vi "IP_Simulation.vi"(8 "error constant":errorcluster, 10 "Enum":T5, 11 "IP_UI":T4) -> (0 "error constant":errorcluster, 3 "Out":T4)   [LabVIEW 2021]
uses:
  Controls/IP_Cellular Tech Type def.ctl
  Controls/IP_Network_Type def.ctl
  Controls/IP_Type-Tydedef.ctl
  APIs/Controls/Base_Station_Emulator.ctl
  Controls/Enum-TypeDef.ctl
panel:
  in  "Base Station":T6
  # "Type"
  # "Network"
  # "Tech"
  # "Client Address"
  # "Throughput (Mbps)"
  # "Duration"
  # "Actions"
  # "IP-SIMULATION"
  # "ASDFADFAF"
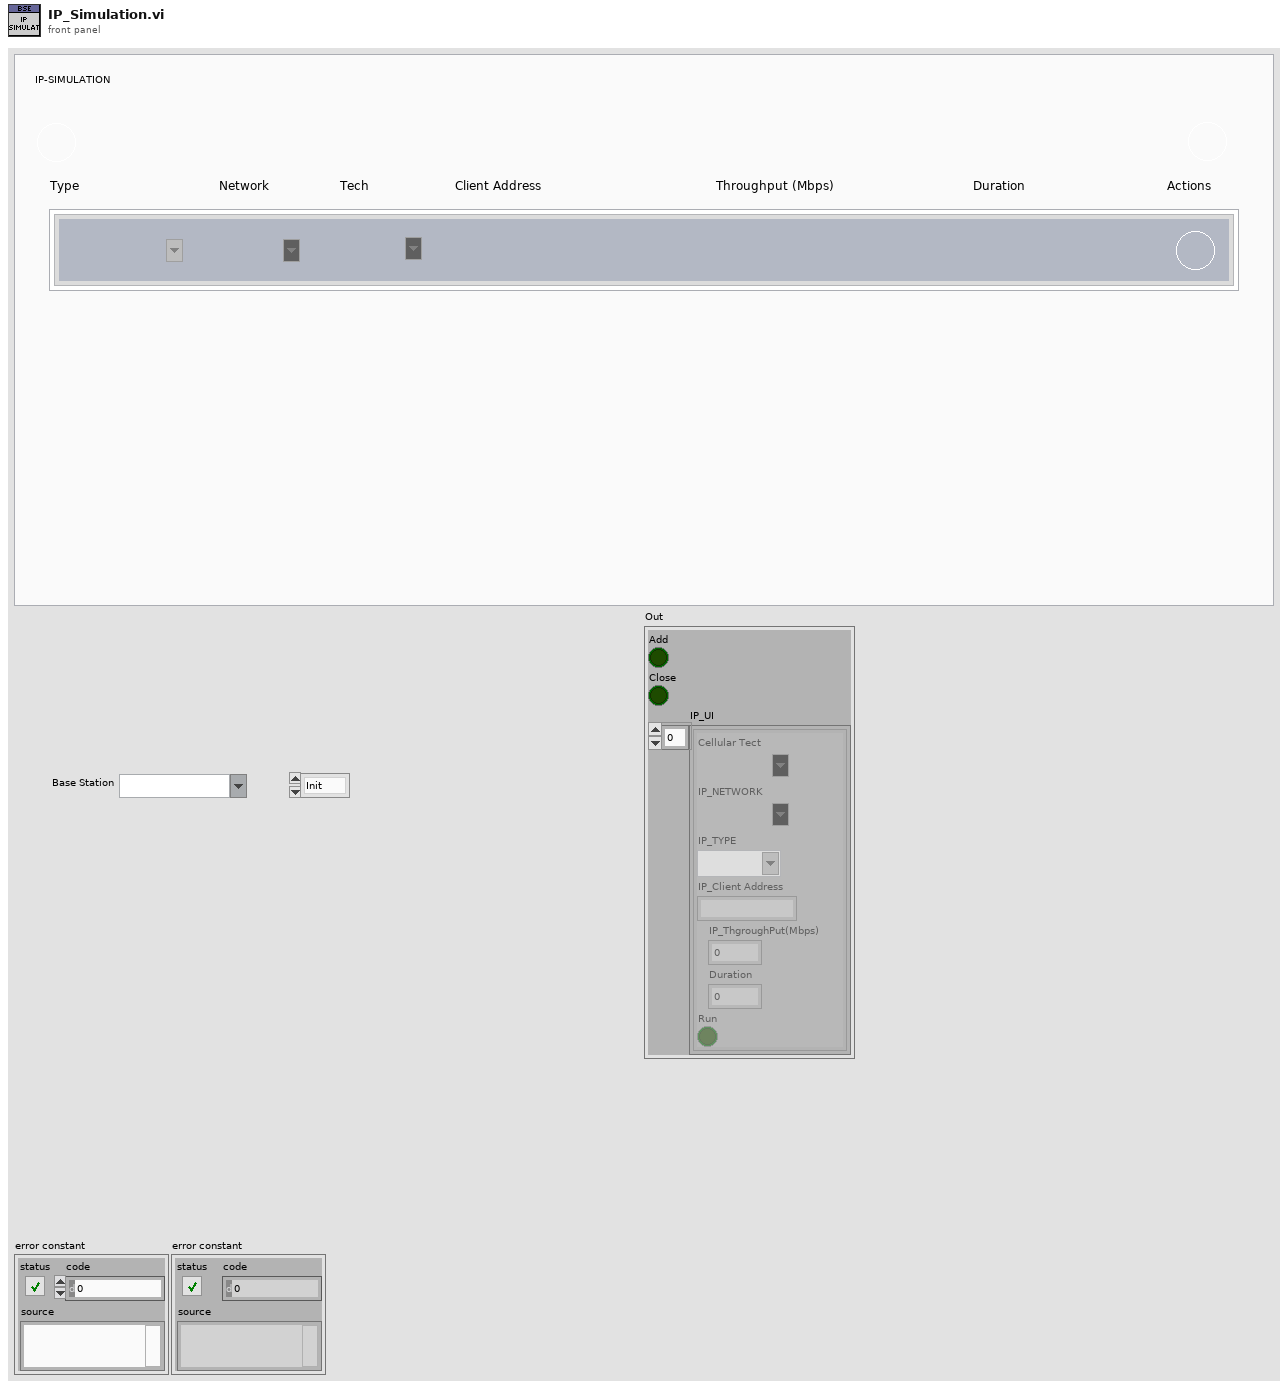
[diagram p1: front panel]
types:
  T1 = typedef "IP_Cellular Tech Type def.ctl" = string
  T2 = typedef "IP_Network_Type def.ctl" = string
  T3 = typedef "IP_Type-Tydedef.ctl" = string
  T4 = cluster{"Add":bool, "Close":bool, "IP_UI":cluster{"Cellular Tect":T1, "IP_NETWORK":T2, "IP_TYPE":T3, "IP_Client Address":string, "IP_ThgroughPut(Mbps)":i32, "Duration":i32, "Run":bool}[]}
  T5 = typedef "Enum-TypeDef.ctl" = enum16{"Init", "poll", "Close"}
  T6 = typedef "Base_Station_Emulator.ctl" = string
  T7 = cluster{"Cellular Tect":T1, "IP_NETWORK":T2, "IP_TYPE":T3, "IP_Client Address":string, "IP_ThgroughPut(Mbps)":i32, "Duration":i32, "Run":bool}[]
  T8 = cluster{"Cellular Tect":T1, "IP_NETWORK":T2, "IP_TYPE":T3, "IP_Client Address":string, "IP_ThgroughPut(Mbps)":i32, "Duration":i32, "Run":bool}
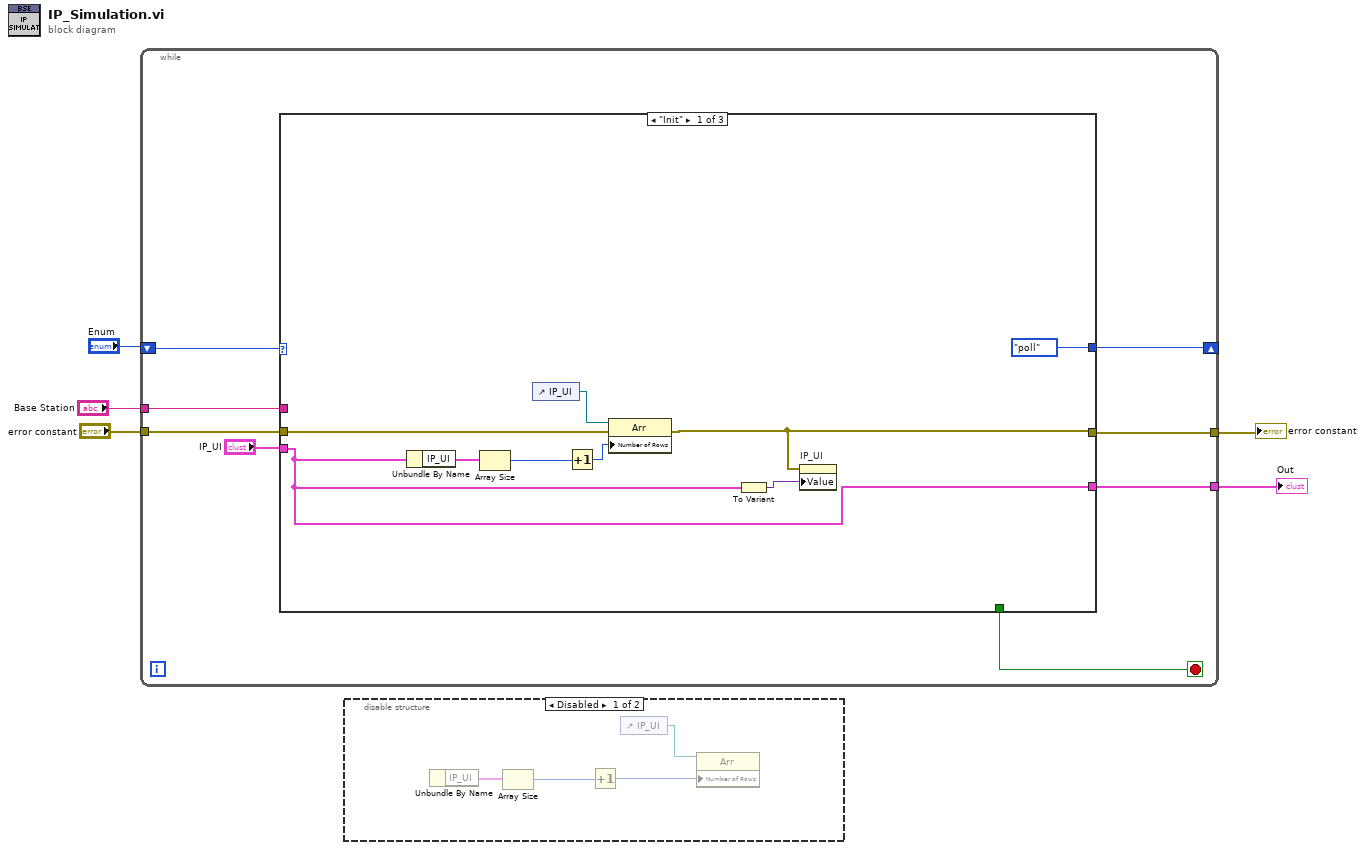
[diagram p0: block diagram]
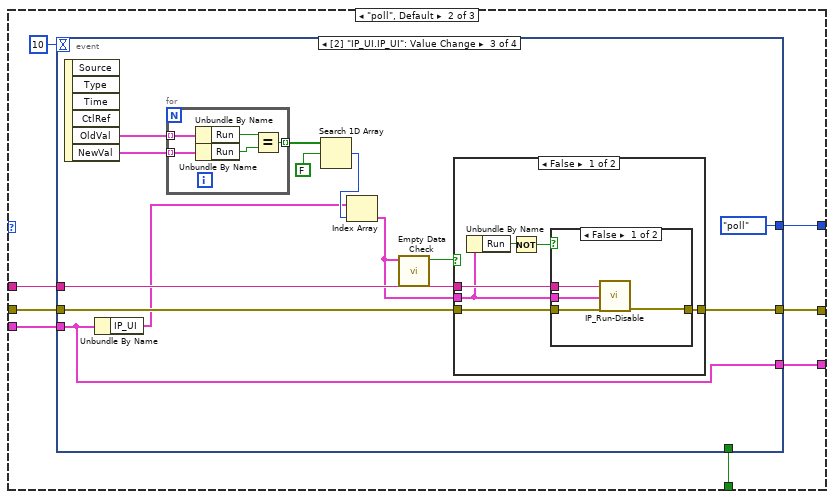
[diagram p3: hidden frame]
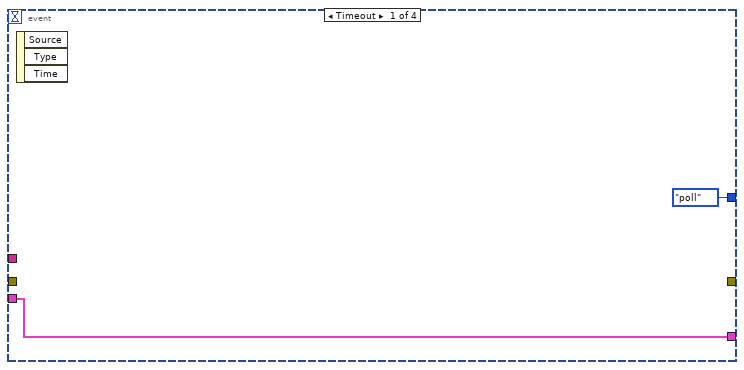
[diagram p4: hidden frame]
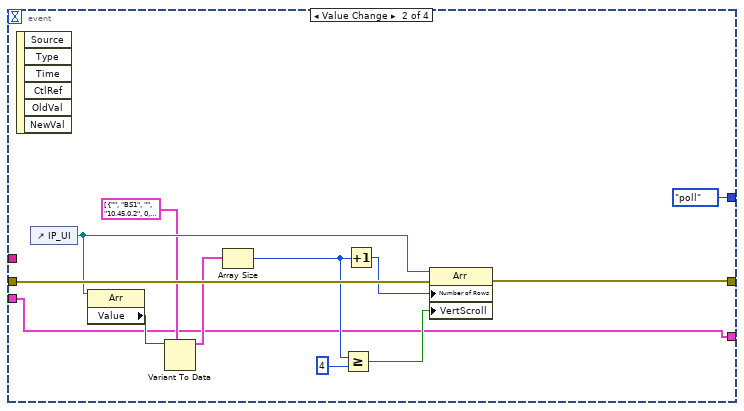
[diagram p5: hidden frame]
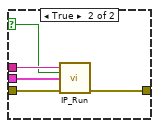
[diagram p6: hidden frame]
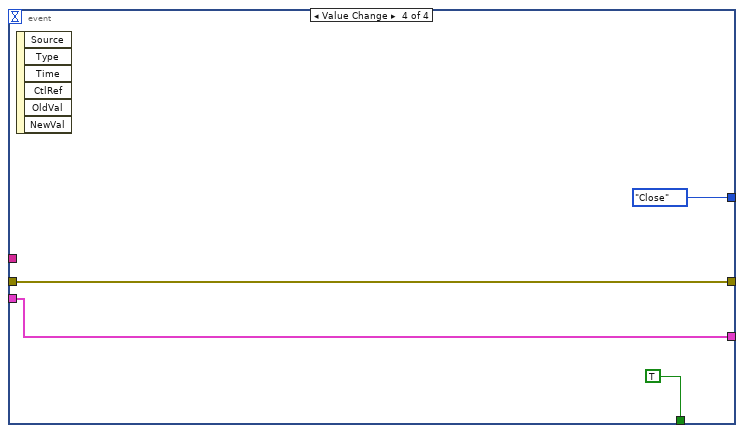
[diagram p8: hidden frame]
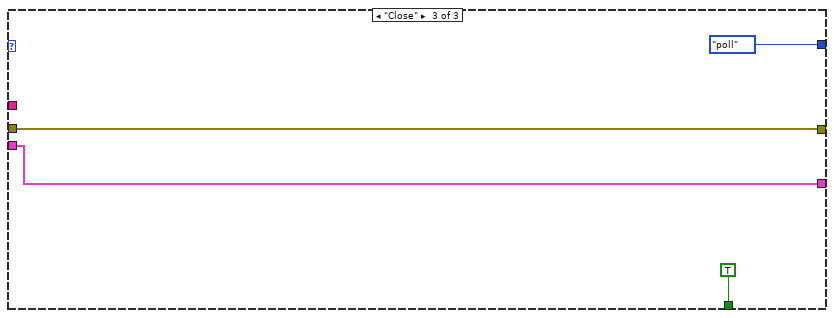
[diagram p9: hidden frame]
diagram:
  n1 = while {
    shift-right: [w11] -> _
    shift-left: "Enum" -> [w12]
    tunnel: "error constant" -> [w10]
    tunnel: [w9] -> w2
    tunnel: "Base Station" -> [w7]
    tunnel: [w6] -> w1
    stop <- w13 stop-if-true
    n2 = case shown="\"Init\"" w12 {
      tunnel: [_ w23 TRUE] -> w13
      tunnel: [Enum-TypeDef."poll" w28 Enum-TypeDef."poll"] -> w11
      tunnel: w10 -> [w21 w30 w85]
      tunnel: [w19 w29 w85] -> w9
      tunnel: "IP_UI" -> [w14 w26 w83]
      tunnel: w7 -> [_ w25 _]
      tunnel: [w14 w24 w83] -> w6
      frame "Init" {
        n3 = Unbundle By Name(w14) -> ("IP_UI"=w17:T7)
        n4 = Array Size(array=w17) -> (size(s)=w16:i32)
        n5 = control-ref of="IP_UI"() -> (w18:refnum<vi>)
        n6 = Increment(x=w16) -> (x+1=w15:i32)
        n7 = property class="Arr"(reference=w18, error in=w21, "Number of Rows"=w15) -> (error out=w19:errorcluster)  [unwired: 1 out]
        n8 = To Variant(anything=w14) -> (Variant=w20:variant)
        n9 = property on="IP_UI" class="Clust"(error in=w19, "Value"=w20) -> ()  [unwired: 1 in, 2 out]
      }
      frame "poll", Default {
        n10 = event shown="[2] \"IP_UI.IP_UI\": Value Change" {
          selector: _ -> [_ _ _ _]
          dyn-events: _ -> [_ _ _ _]
          timeout: 10 -> [_ _ _ _]
          tunnel: w30 -> [_ w44 w54 w81]
          tunnel: [_ w39 w53 w81] -> w29
          tunnel: [Enum-TypeDef."poll" Enum-TypeDef."poll" Enum-TypeDef."poll" Enum-TypeDef."Close"] -> w28
          tunnel: w25 -> [_ _ w52 _]
          tunnel: w26 -> [w31 w33 w45 w80]
          tunnel: [w31 w33 w45 w80] -> w24
          tunnel: [_ _ _ TRUE] -> w23
          event Timeout {
            n11 = event-data() -> ()  [unwired: 1 in, 3 out]
          }
          event "IP_UI.Add": Value Change {
            n12 = event-data() -> ()  [unwired: 1 in, 6 out]
            n13 = control-ref of="IP_UI"() -> (w37:refnum<vi>)
            n14 = property class="Arr"(reference=w37) -> ("Value"=w36:variant)  [unwired: 1 in, 2 out]
            n15 = Variant To Data(type=T7 [{"Cellular Tect"="", "IP_NETWORK"="BS1", "IP_TYPE"="", "IP_Client Address"="10.45.0.2", "IP_ThgroughPut(Mbps)"=0, "Duration"=0, "Run"=FALSE}] ("IP_UI"), Variant=w36) -> (data=w34:T7)  [unwired: 1 in, 1 out]
            n16 = Array Size(array=w34) -> (size(s)=w42:i32)
            n17 = Greater Or Equal?(x=w42, y=4) -> (x >= y?=w40:bool)
            n18 = Increment(x=w42) -> (x+1=w38:i32)
            n19 = property class="Arr"(reference=w37, error in=w44, "Number of Rows"=w38, "VertScroll"=w40) -> (error out=w39:errorcluster)  [unwired: 1 out]
          }
          event "IP_UI.IP_UI": Value Change {
            n20 = event-data() -> ("OldVal"=w49:T7, "NewVal"=w57:T7)  [unwired: 1 in, 4 out]
            n21 = Unbundle By Name(w45) -> ("IP_UI"=w48:T7)
            n22 = for {
              tunnel: w49 -> [w77] mode=indexing
              tunnel: w57 -> [w78] mode=indexing
              tunnel: [w76] -> w50 mode=indexing
              n23 = Unbundle By Name(w77) -> ("Run"=w74:bool)
              n24 = Unbundle By Name(w78) -> ("Run"=w75:bool)
              n25 = Equal?(x=w74, y=w75) -> (x = y?=w76:bool)
            }
            n26 = Search 1D Array(1D array=w50, element=FALSE) -> (index of element=w56:i32)  [unwired: 1 in]
            n27 = Index Array(array=w48, index=w56) -> (element=w47:T8)
            n28 = call "Empty Data Check.vi"("Cluster Data"=w47) -> ("Empty?"=w46:bool)  [unwired: 10 in]
            n29 = case shown="False" w46 {
              tunnel: w54 -> [w63 w73]
              tunnel: [w62 w73] -> w53
              tunnel: w52 -> [w61 _]
              tunnel: w47 -> [w58 _]
              frame False {
                n30 = Unbundle By Name(w58) -> ("Run"=w60:bool)
                n31 = Not(x=w60) -> (.not. x?=w59:bool)
                n32 = case shown="False" w59 {
                  selector: w59 -> [_ w68]
                  tunnel: w58 -> [w64 w69]
                  tunnel: w63 -> [w67 w72]
                  tunnel: [w66 w71] -> w62
                  tunnel: w61 -> [w65 w70]
                  frame False {
                    n33 = call "IP_Run-Disable.vi"("Base Station"=w65, "Element"=w64, "error in (no error)"=w67) -> ("error out"=w66:errorcluster)  [unwired: 11 in, 1 out]
                  }
                  frame True {
                    n34 = call "IP_Run.vi"("Base Station"=w70, "Status"=w68, "Element"=w69, "error in (no error)"=w72) -> ("error out"=w71:errorcluster)  [unwired: 11 in]
                  }
                }
              }
              frame True {
              }
            }
          }
          event "IP_UI.Close": Value Change {
            n35 = event-data() -> ()  [unwired: 1 in, 6 out]
          }
        }
      }
      frame "Close" {
      }
    }
  }
  "error constant" <- w2
  "Out" <- w1
  n36 = disable-structure shown="Disabled" {
    frame Disabled {
      n37 = Unbundle By Name() -> ("IP_UI"=w88:T7)  [unwired: 1 in]
      n38 = Array Size(array=w88) -> (size(s)=w89:i32)
      n39 = Increment(x=w89) -> (x+1=w90:i32)
      n40 = control-ref of="IP_UI"() -> (w87:refnum<vi>)
      n41 = property class="Arr"(reference=w87, "Number of Rows"=w90) -> ()  [unwired: 1 in, 2 out]
    }
    frame Enabled {
    }
  }
